vi "Transfer Controller.vi"(8 "error in":errorcluster) -> ()   [LabVIEW 2023]
doc: "This VI executes continuously carrying out the current operation and responding to updates or new operations. It will often contain the timing or control code that is difficult to place directly in TeleOp. This VI generally opens all sensors and motors and isolates the rest of the robot code from knowing how the operations are carried out."
uses:
  <vilib>/Rock Robotics/WPI/Framework/Completion Status.ctl
  Transfer Setpoints.ctl
  Transfer Operations.ctl
  <vilib>/Rock Robotics/Network Tables/NT Write Boolean.vi
panel:
  in  "Output":dbl=0.8 format="%#_13g"
  in  "Interactive Values":T1
  out "Current\nCmd":string="Started at  19:39:36.614\nDefault: Reserve,  "
  in  "Buttons":cluster{"Execute Cmd":bool, "Abort Cmd":bool}
  out "Command Timing":cluster{"Start Time (ms)":u32, "Iterations":i32}={"Start Time (ms)"=1307604, "Iterations"=0}
  out "Status":T3
  # "Tip: It may be helpful to observe inputs and sensor values.\nYou may also want to display tuning or debugging controls."
  # "Interactive Command: You may fill in the settings for a command\nand schedule it with the Execute button. You can observe and abort\nany command while fine tuning the code for the controller."
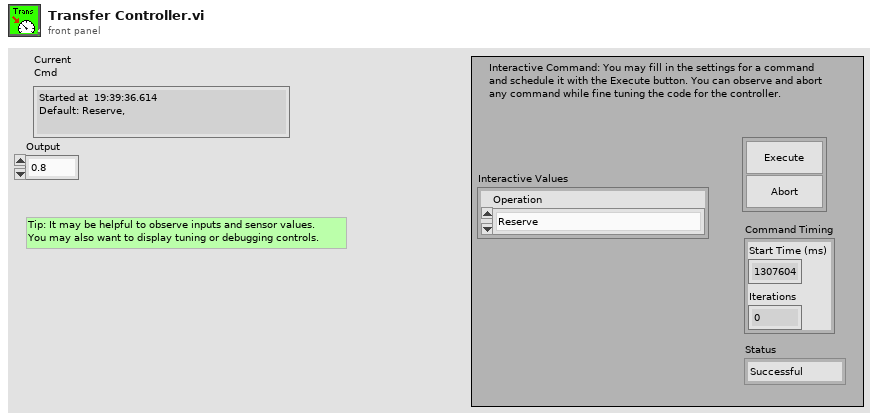
[diagram p1: front panel]
types:
  T1 = typedef "Transfer Setpoints.ctl" = cluster{"Operation":T2}
  T2 = typedef "Transfer Operations.ctl" = enum16{"Reserve", "Read Current", "Immediate", "On", "Off", "Reject"}
  T3 = typedef "Completion Status.ctl" = enum16{"Successful", "Aborted", "Incomplete"}
  T4 = typedef "Command Status Info.ctl" = cluster{"Name":string, "Status":T3, "notifier out":T5}
  T5 = typedef "Completion Notifier.ctl" = refnum<notifier>
  T6 = cluster{"Current Command":T1, "Command Timing":cluster{"Start Time (ms)":u32, "Iterations":i32}, "Command Arguments":cluster{"Command Info":T4, "Description":string, "Default Command":T1, "queue out":refnum<queue>, "Subsystem Name":string}}
  T7 = typedef "Color Sensor V3 DevRef.ctl" = cluster{"I2CDevRef":T8}
  T8 = typedef "WPI_I2CDevRef.ctl" = cluster{"DevStatus":errorcluster, "Device Address":u8, "Handle":i32, "I2C Bus":T9}
  T9 = typedef "i2c_bus.ctl" = enum16{"I2C On-Board", "I2C MXP", "Invalid"}
  T10 = typedef "WPI_MotorControlDeviceRef.ctl" = cluster{"DeviceStatus":errorcluster, "Type":T11, "PWM":cluster{"PWM Channel":T12, "DeadBand":T13}, "CAN":cluster{"Device Number":u8, "SetOutput VI Ref":variant, "GetOutput VI Ref":variant, "Enable VI Ref":variant, "Disable VI Ref":variant, "Data":variant}, "Invert":bool, "DIO PWM":cluster{"PWM \"Enable\" Channel":T12, "DIOChannel":T14, "PWM Rate":dbl}}
  T11 = typedef "WPI_MotorControlType.ctl" = enum16{"PWM", "CAN", "DIO PWM"}
  T12 = typedef "FPGA_DIOPWMChannel.ctl" = enum8{"PWM 0", "PWM 1", "PWM 2", "PWM 3", "PWM 4", "PWM 5", "PWM 6", "PWM 7", "PWM 8", "PWM 9", "PWM MXP 0", "PWM MXP 1", "PWM MXP 2", "PWM MXP 3", "PWM MXP 4", "PWM MXP 5", "PWM MXP 6", "PWM MXP 7", "PWM MXP 8", "PWM MXP 9", "Invalid"}
  T13 = typedef "WPI_PWMDeadband.ctl" = cluster{"Name":string, "maxPositivePwm":i32, "minPositivePwm":i32, "centerPwm":i32, "maxNegativePwm":i32, "minNegativePwm":i32, "angularRange":u16}
  T14 = typedef "FPGA_DIOChannel.ctl" = enum8{"DIO 0", "DIO 1", "DIO 2", "DIO 3", "DIO 4", "DIO 5", "DIO 6", "DIO 7", "DIO 8", "DIO 9", "DIO MXP 0", "DIO MXP 1", "DIO MXP 2", "DIO MXP 3", "DIO MXP 4", "DIO MXP 5", "DIO MXP 6", "DIO MXP 7", "DIO MXP 8", "DIO MXP 9", "DIO MXP 10", "DIO MXP 11", "DIO MXP 12", "DIO MXP 13", "DIO MXP 14", "DIO MXP 15", "SPI Port CS1", "SPI Port CS2", "SPI Port CS3", "SPI Port MISO", "SPI Port MOSI", "Invalid"}
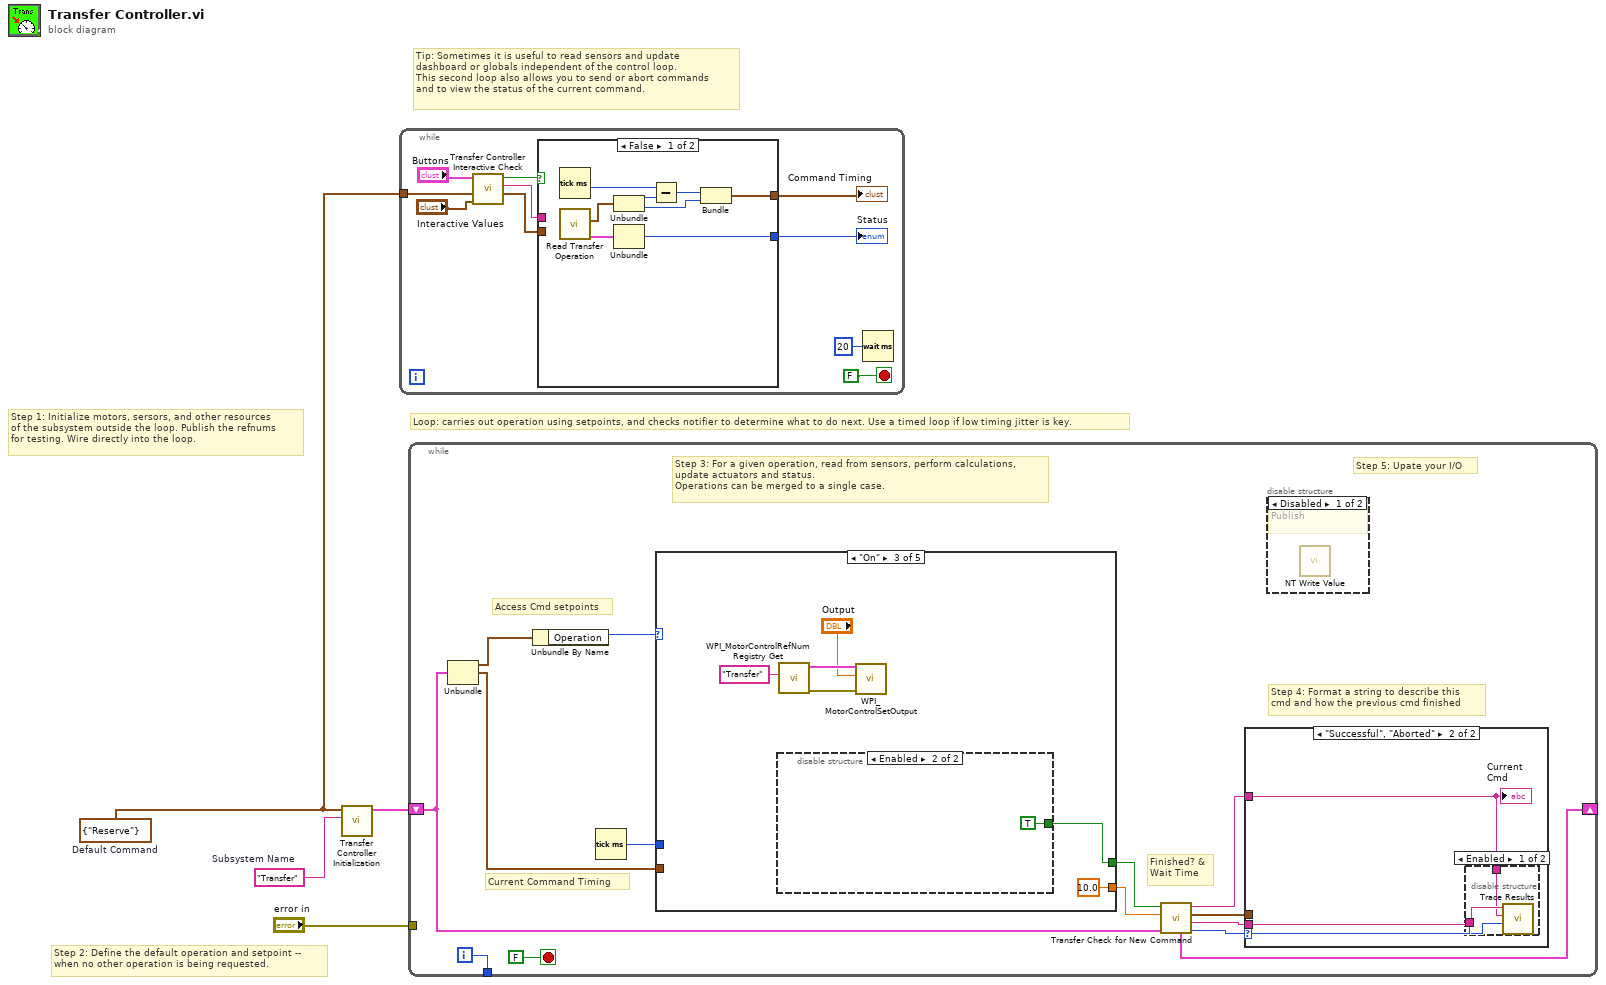
[diagram p0: block diagram]
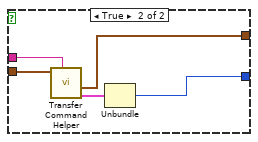
[diagram p2: hidden frame]
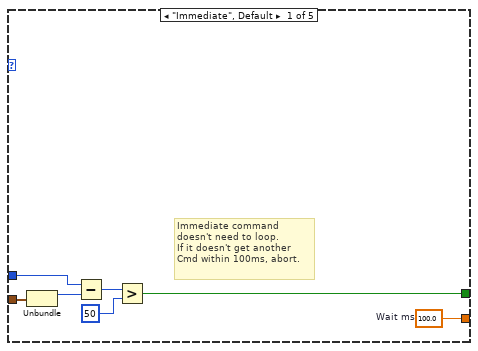
[diagram p6: hidden frame]
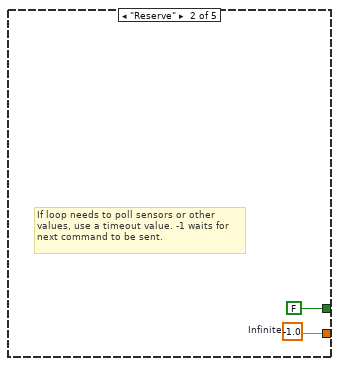
[diagram p7: hidden frame]
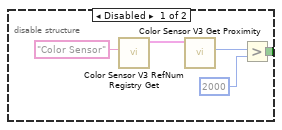
[diagram p8: hidden frame]
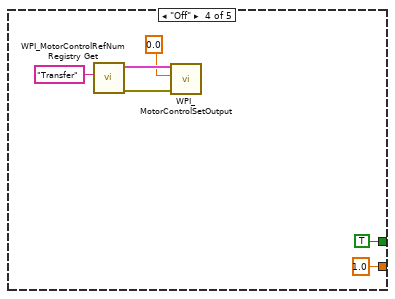
[diagram p9: hidden frame]
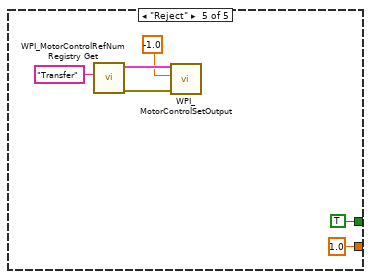
[diagram p10: hidden frame]
diagram:
  w1 = T1 {"Operation"=enum."Reserve"}  # Default Command
  w2 = "Transfer"  # Subsystem Name
  # "Tip: Sometimes it is useful to read sensors and update\ndashboard or globals independent of the control loop.\nThis second loop also allows you to send or abort commands\nand to view the status of the current command."
  # "Step 2: Define the default operation and setpoint --\nwhen no other operation is being requested."
  # "Step 1: Initialize motors, sersors, and other resources\nof the subsystem outside the loop. Publish the refnums\nfor testing. Wire directly into the loop."
  # "Loop: carries out operation using setpoints, and checks notifier to determine what to do next. Use a timed loop if low timing jitter is key."
  n1 = call "Transfer Controller Initialization.vi"("Subsystem Name"=w2, "Default Command"=w1) -> ("Current Command"=w3:T6)  [unwired: 9 in]
  n2 = while {
    tunnel: w1 -> [w11]
    stop <- FALSE stop-if-true
    n3 = call "Transfer Controller Interactive Check.vi"("Interactive Command in"="Interactive Values", "Default Command"=w11, "Buttons"="Buttons") -> ("Interactive Command out"=w8:T1, "Trace String"=w9:string, "Schedule"=w10:bool)  [unwired: 6 in]
    n4 = case shown="False" w10 {
      tunnel: [w22 w27] -> w7
      tunnel: w8 -> [_ w25]
      tunnel: [w15 w23] -> w6
      tunnel: w9 -> [_ w26]
      frame False {
        n5 = Tick Count (ms)() -> (millisecond timer value=w18:u32)
        n6 = call "Read Transfer Operation.vi"() -> ("Command Info"=w17:T4, "Command Timing"=w16:cluster{"Start Time (ms)":u32, "Iterations":i32})  [unwired: 9 in, 1 out]
        n7 = Unbundle(w16) -> ("Start Time (ms)"=w21:u32, "Iterations"=w19:i32)
        n8 = Unbundle(w17) -> ("Status"=w22:T3)  [unwired: 2 out]
        n9 = Subtract(x=w18, y=w21) -> (x-y=w20:u32)
        n10 = Bundle(w20, "Iterations"=w19) -> (w15:cluster{u32, "Iterations":i32})  [unwired: 1 in]
      }
      frame True {
        n11 = call "Transfer Command Helper.vi"("Description"=w26, "SubSystem Data"=w25) -> ("Command Info Out"=w24:T4, "Command Timing"=w23:cluster{"Start Time (ms)":u32, "Iterations":i32})  [unwired: 7 in, 1 out]
        n12 = Unbundle(w24) -> ("Status"=w27:T3)  [unwired: 2 out]
      }
    }
    "Status" <- w7
    "Command Timing" <- w6
    n13 = Wait (ms)(milliseconds to wait=u32 20) -> ()  [unwired: 1 out]
  }
  n14 = while {
    shift-right: [w35] -> _
    shift-left: w3 -> [w28]
    tunnel: [w40] -> _
    tunnel: "error in" -> [_]
    i -> [w40]
    stop <- FALSE stop-if-true
    # "Step 5: Upate your I/O"
    # "Step 4: Format a string to describe this\ncmd and how the previous cmd finished"
    # "Current Command Timing"
    # "Access Cmd setpoints"
    # "Finished? &\nWait Time"
    # "Step 3: For a given operation, read from sensors, perform calculations,\nupdate actuators and status.\nOperations can be merged to a single case."
    n15 = Unbundle(w28) -> ("Current Command"=w39:T1, "Command Timing"=w36:cluster{"Start Time (ms)":u32, "Iterations":i32})  [unwired: 1 out]
    n16 = Unbundle By Name(w39) -> ("Operation"=w38:T2)
    n17 = Tick Count (ms)() -> (millisecond timer value=w37:u32)
    n18 = case shown="\"On\"" w38 {
      tunnel: [w54 w56 10.0 ("Infinite") 1.0 ("Infinite") 1.0 ("Infinite")] -> w33
      tunnel: [w48 FALSE ("ignore previous (F)") w57 TRUE ("ignore previous (F)") TRUE ("ignore previous (F)")] -> w34
      tunnel: w36 -> [w50 _ _ _ _]
      tunnel: w37 -> [w49 _ _ _ _]
      frame "Immediate", Default {
        w54 = 100.0  # Wait ms
        # "Immediate command\ndoesn't need to loop.\nIf it doesn't get another\nCmd within 100ms, abort."
        n19 = Unbundle(w50) -> ("Start Time (ms)"=w53:u32)  [unwired: 1 out]
        n20 = Subtract(x=w49, y=w53) -> (x-y=w52:u32)
        n21 = Greater?(x=w52, y=u8 50 ("Left Motor")) -> (0:w48:bool)
      }
      frame "Reserve" {
        w56 = -1.0  # Infinite
        # "If loop needs to poll sensors or other\nvalues, use a timeout value. -1 waits for\nnext command to be sent."
      }
      frame "On" {
        n22 = disable-structure shown="Enabled" {
          disable-tunnel: [w63 TRUE] -> w57
          frame Disabled {
            n23 = call <vilib>:"Color Sensor V3 RefNum Registry Get.vi"("refnum name"="Color Sensor") -> ("ColorSensorDevRef"=w67:T7)  [unwired: 9 in, 1 out]
            n24 = call <vilib>:"Color Sensor V3 Get Proximity.vi"("ColorSensorDevRef"=w67) -> ("Proximity"=w65:u16)  [unwired: 8 in, 2 out]
            n25 = Greater?(x=w65, y=u16 2000) -> (0:w63:bool)
          }
          frame Enabled {
          }
        }
        n26 = call <vilib>:"WPI_MotorControlRefNum Registry Get.vi"("refnum name"="Transfer") -> ("error out"=w61:errorcluster, "MotorControlDevRef"=w60:T10)  [unwired: 9 in]
        n27 = call <vilib>:"WPI_MotorControlSetOutput.vi"("error in (no error)"=w61, "Output"="Output", "MotorControlDevRef"=w60) -> ()  [unwired: 6 in, 3 out]
      }
      frame "Off" {
        n28 = call <vilib>:"WPI_MotorControlRefNum Registry Get.vi"("refnum name"="Transfer") -> ("error out"=w73:errorcluster, "MotorControlDevRef"=w72:T10)  [unwired: 9 in]
        n29 = call <vilib>:"WPI_MotorControlSetOutput.vi"("error in (no error)"=w73, "Output"=0.0, "MotorControlDevRef"=w72) -> ()  [unwired: 6 in, 3 out]
      }
      frame "Reject" {
        n30 = call <vilib>:"WPI_MotorControlRefNum Registry Get.vi"("refnum name"="Transfer") -> ("error out"=w79:errorcluster, "MotorControlDevRef"=w78:T10)  [unwired: 9 in]
        n31 = call <vilib>:"WPI_MotorControlSetOutput.vi"("error in (no error)"=w79, "Output"=-1.0, "MotorControlDevRef"=w78) -> ()  [unwired: 6 in, 3 out]
      }
    }
    n32 = call "Transfer Check for New Command.vi"("Current Command"=w28, "Wait time (ms)"=w33, "Finished?"=w34) -> ("Completion"=w29:T3, "Subsystem Name"=w30:string, "Current Command"=w31:T1, "Initial Trace String"=w32:string, "NextCommand"=w35:T6)  [unwired: 4 in]
    n33 = case shown="\"Successful\", \"Aborted\"" w29 {
      selector: w29 -> [_ w44]
      tunnel: w32 -> [_ w42]
      tunnel: w31 -> [_ _]
      tunnel: w30 -> [_ w43]
      frame "Incomplete", Default {
        # "Continuing current command"
      }
      frame "Successful", "Aborted" {
        # "Report and setup for next command"
        n34 = disable-structure shown="Enabled" {
          disable-tunnel: w44 -> [w47 _]
          disable-tunnel: w43 -> [w46 _]
          disable-tunnel: w42 -> [w45 _]
          frame Enabled {
            n35 = call <vilib>:"Trace Results.vi"("Status of previous command"=w47, "Description"=w45, "Subsystem"=w46) -> ()  [unwired: 9 in]
          }
          frame Disabled {
          }
        }
        "Current\nCmd" <- w42
      }
    }
    n36 = disable-structure shown="Disabled" {
      frame Disabled {
        # "Publish"
        n37 = call-poly <vilib>:"NT Write Value.vi"() -> ()  [unwired: 11 in, 1 out]
      }
      frame Enabled {
      }
    }
  }
